vi "merge_Pulse Timer.vi"   [LabVIEW 2017, in "NI_FunctionBlockMergeVIs.lvlib"]
doc: "Generates output pulses triggered by rising edges on the <B>input</B> signal."
uses:
  <vilib>/functionblocks/NI_FunctionBlockMergeVIs.lvlib
  <vilib>/functionblocks/FB Core/FB Core.xnode
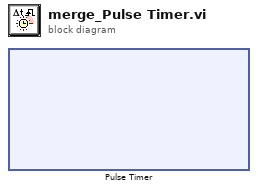
[diagram p0: block diagram]
diagram:
  n1 = xnode "Pulse Timer"() -> ()  [unwired: 3 in, 3 out]
